vi "weahter.vi"() -> ()   [LabVIEW 2021]
uses:
  <vilib>/Utility/NIReport.llb/NI_report.lvclass
  <vilib>/httpClient/LabVIEWHTTPClient.lvlib
panel:
  in  "Закрыть":bool
  out "Погода 2":picture
  out "Город":picture
  in  "Город n":string(combo)
  out "Кластер погоды":T1
  in  "Кластер погоды 1":T1
  out "body":string
  # "Координаты"
  # "Закат"
  # "Рассвет"
  # "Температура, К"
  # "Ощущается как"
  # "Влажность"
  # "Давление"
  # "Долгота"
  # "Широта"
  # "Координаты"
  # "Закат"
  # "Рассвет"
  # "Температура, К"
  # "Ощущается как"
  # "Влажность"
  # "Давление"
  # "Долгота"
  # "Широта"
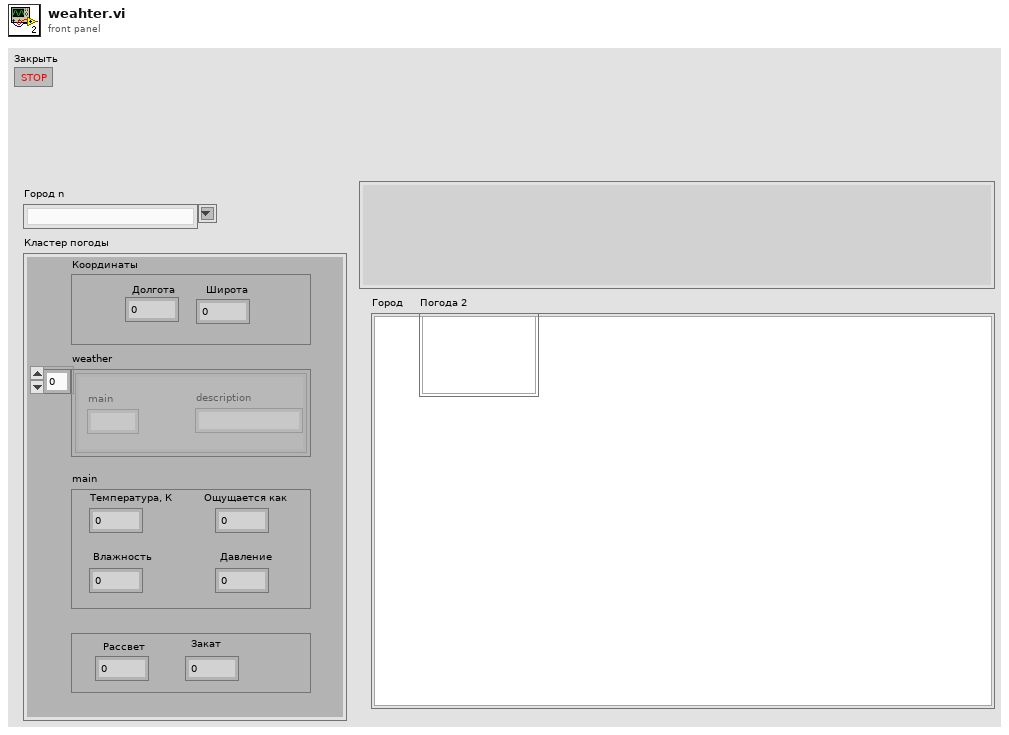
[diagram p1: front panel]
types:
  T1 = typedef "Кластер погоды.ctl" = cluster{"coord":cluster{"lon":dbl, "lat":dbl}, "weather":cluster{"main":string, "description":string}[], "main":cluster{"temp":dbl, "feels_like":dbl, "pressure":dbl, "humidity":dbl}, "sys":cluster{"sunrise":dbl, "sunset":dbl}}
  T2 = enum16{"Standard Report", "HTML", "Word", "Excel"}
  T3 = typedef "imagedata.ctl" = cluster{"image type":i32, "image depth":i32, "image":u8[], "mask":u8[], "colors":u32[], "Rectangle":cluster{"left":i16, "top":i16, "right":i16, "bottom":i16}}
  T4 = cluster{"temp":dbl, "feels_like":dbl, "pressure":dbl, "humidity":dbl}
  T5 = cluster{"weather[0]":cluster{"main":string, "description":string}, "weather[1]":cluster{"main":string, "description":string}, "weather[2]":cluster{"main":string, "description":string}, "weather[3]":cluster{"main":string, "description":string}, "weather[4]":cluster{"main":string, "description":string}, "weather[5]":cluster{"main":string, "description":string}, "weather[6]":cluster{"main":string, "description":string}, "weather[7]":cluster{"main":string, "description":string}, "weather[8]":cluster{"main":string, "description":string}}
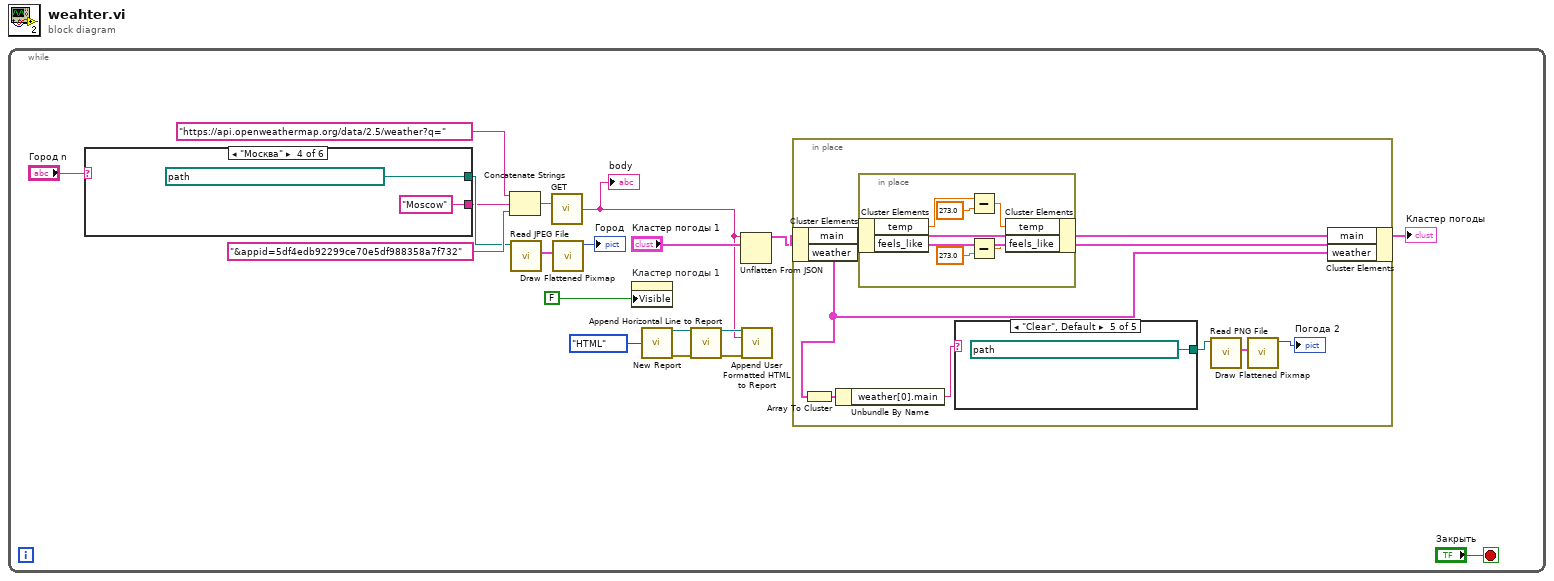
[diagram p0: block diagram]
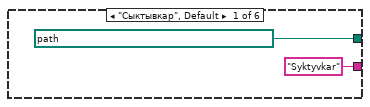
[diagram p2: hidden frame]
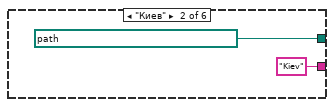
[diagram p3: hidden frame]
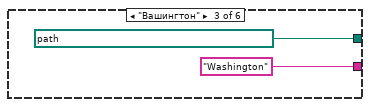
[diagram p4: hidden frame]
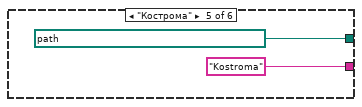
[diagram p5: hidden frame]
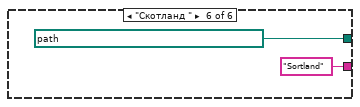
[diagram p6: hidden frame]
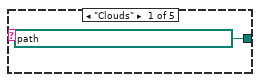
[diagram p7: hidden frame]
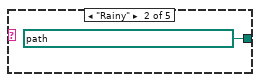
[diagram p8: hidden frame]
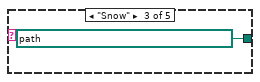
[diagram p9: hidden frame]
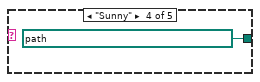
[diagram p10: hidden frame]
diagram:
  n1 = while {
    stop <- "Закрыть" stop-if-true
    n2 = case shown="\"Москва\"" "Город n" {
      tunnel: ["Syktyvkar" ("url") "Kiev" ("url") "Washington" ("url") "Moscow" ("url") "Kostroma" ("url") "Sortland" ("url")] -> w2
      tunnel: [path "D:/8sem/LabView/Погода/Сыктывкар.jpg" ("path to PNG file") path "D:/8sem/LabView/Погода/Киев.jpg" ("path to PNG file") path "D:/8sem/LabView/Погода/Вашингтон.jpg" ("path to PNG file") path "D:/8sem/LabView/Погода/Москва.jpg" ("path to PNG file") path "D:/8sem/LabView/Погода/Кострома.jpg" ("path to PNG file") path "D:/8sem/LabView/Погода/Скотланд.jpg" ("path to PNG file")] -> w3
      frame "Сыктывкар", Default {
      }
      frame "Киев" {
      }
      frame "Вашингтон" {
      }
      frame "Москва" {
      }
      frame "Кострома" {
      }
      frame "Скотланд " {
      }
    }
    n3 = Concatenate Strings("https://api.openweathermap.org/data/2.5/weather?q=" ("url"), w2, "&appid=5df4edb92299ce70e5df988358a7f732" ("url")) -> (w12:string)
    n4 = call <vilib>:"Read JPEG File.vi"("path to JPEG file"=w3) -> ("image data"=w6:T3)  [unwired: 8 in, 2 out]
    n5 = call <vilib>:"GET.vi"("url"=w12) -> ("body"=w4:string)  [unwired: 11 in, 3 out]
    "body" <- w4
    n6 = call <vilib>:"Draw Flattened Pixmap.vi"("image data"=w6) -> ("new picture"=→"Город":picture)  [unwired: 8 in]
    n7 = property on="Кластер погоды 1" class="Clust (strict)"("Visible"=FALSE) -> ()  [unwired: 2 in, 2 out]
    n8 = call <vilib>:"New Report.vi"("report type"=T2."HTML") -> ("report out"=w18:refnum<class "NI_report.lvclass">, "error out"=w17:errorcluster)  [unwired: 13 in]
    n9 = call-dynamic "Append Horizontal Line to Report.vi"("report in"=w18, "error in (no error)"=w17) -> ("report out"=w16:refnum<class "NI_report.lvclass">, "error out"=w15:errorcluster)  [unwired: 12 in]
    n10 = Unflatten From JSON(JSON string=w4, type and defaults="Кластер погоды 1") -> (value=w5:T1)  [unwired: 5 in, 1 out]
    n11 = call-dynamic "Append User Formatted HTML to Report.vi"("report in"=w16, "HTML text"=w4, "error in (no error)"=w15) -> ()  [unwired: 11 in, 2 out]
    n12 = in-place {
      n13 = in-place-cluster #1(w5) -> ("main"=w39:T4, "weather"=w35:cluster{"main":string, "description":string}[])
      n14 = Array To Cluster(array=w35) -> (cluster=w36:T5)
      n15 = Unbundle By Name(w36) -> ("weather[0].main"=w37:string)
      n16 = in-place {
        n17 = in-place-cluster #2(w39) -> ("temp"=w48:dbl, "feels_like"=w47:dbl)
        n18 = Subtract(x=w48, y=273.0) -> (x-y=w46:dbl)
        n19 = Subtract(x=w47, y=273.0) -> (x-y=w45:dbl)
        n20 = in-place-cluster #2("temp"=w46, "feels_like"=w45) -> (w38:T4)
      }
      n21 = case shown="\"Clear\", Default" w37 {
        tunnel: [path "D:/8sem/LabView/Погода/Clouds.png" ("path to PNG file") path "D:/8sem/LabView/Погода/Rainy.png" ("path to PNG file") path "D:/8sem/LabView/Погода/Snowy.png" ("path to PNG file") path "D:/8sem/LabView/Погода/Sunny.jpg" ("path to PNG file") path "D:/8sem/LabView/Погода/Clear.png" ("path to PNG file")] -> w32
        frame "Clouds" {
        }
        frame "Rainy" {
        }
        frame "Snow" {
        }
        frame "Sunny" {
        }
        frame "Clear", Default {
        }
      }
      n22 = call <vilib>:"Read PNG File.vi"("path to PNG file"=w32) -> ("image data"=w33:T3)  [unwired: 8 in, 2 out]
      n23 = call <vilib>:"Draw Flattened Pixmap.vi"("image data"=w33) -> ("new picture"=→"Погода 2":picture)  [unwired: 8 in]
      n24 = in-place-cluster #1("main"=w38, "weather"=w35) -> (→"Кластер погоды":T1)
    }
  }
